vi "GXML Versioning.vi"() -> ()   [LabVIEW 2009]
doc: "This example demonstrates how to implement versioning with GXML."
uses:
  _subVIis/GXML SearchParser/gxml_SearchParser.vi
panel:
  out "Config Info v2.0":T1
  out "XML String Out":string
  in  "ConfigInfo v1.0":T2={"Enable"=TRUE, "Sample Rate"=51200.0, "Description"="Acquisition 1"}
  # "This example shows how an application can use GXML versioning to determine which type definition should be used to parse the XML string and how data from older versions can be updated to the current version.\n\nIn this example a configuration is written using an older cluster type definition (version 1.0).  The consuming\napplication however is expecting to parse its data using the current type definition (version 2.0)."
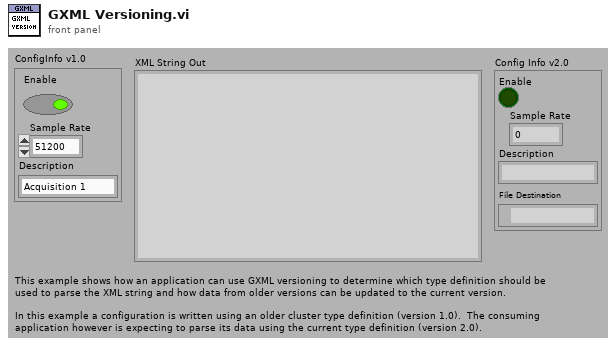
[diagram p1: front panel]
types:
  T1 = cluster{"Enable":bool, "Sample Rate":dbl, "Description":string, "File Destination":path}
  T2 = cluster{"Enable":bool, "Sample Rate":dbl, "Description":string}
  T3 = cluster{"Enable":bool, "Sample Rate":dbl, "Description":string, "Path":path}
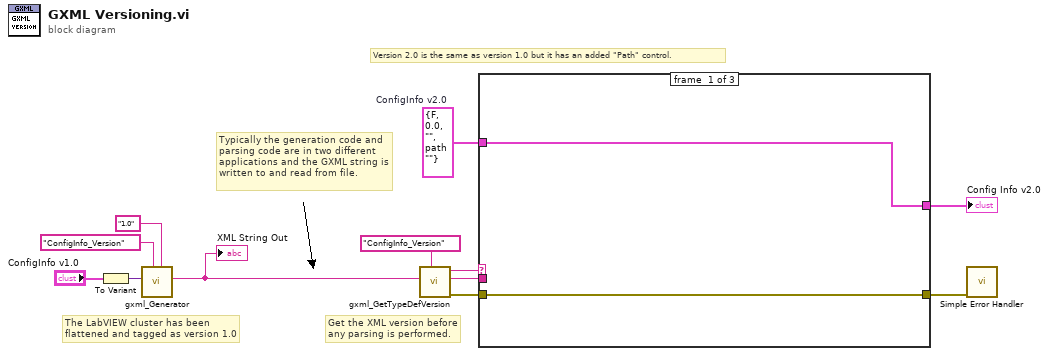
[diagram p0: block diagram]
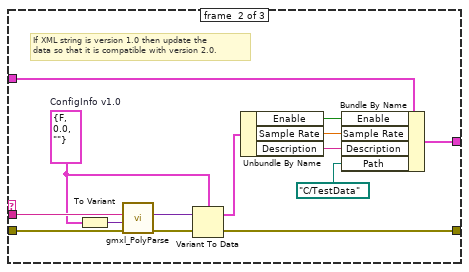
[diagram p2: hidden frame]
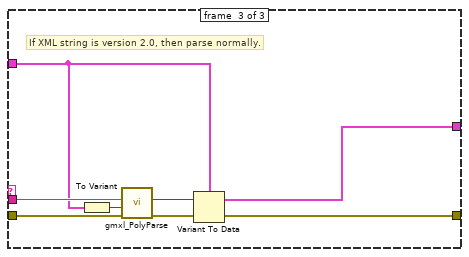
[diagram p3: hidden frame]
diagram:
  w5 = T3 {"Enable"=FALSE, "Sample Rate"=0.0, "Description"="", "Path"=path ""}  # ConfigInfo v2.0
  # "Typically the generation code and parsing code are in two different applications and the GXML string is written to and read from file."
  # "The LabVIEW cluster has been\nflattened and tagged as version 1.0"
  # "Get the XML version before\nany parsing is performed."
  # "Version 2.0 is the same as version 1.0 but it has an added \"Path\" control."
  n1 = To Variant(anything="ConfigInfo v1.0") -> (Variant=w9:variant)
  n2 = call "gxml_Generator.vi"("Version String"="1.0", "Version Tag Name"="ConfigInfo_Version", "Variant"=w9) -> ("XML String Out"=w1:string)  [unwired: 7 in, 1 out]
  "XML String Out" <- w1
  n3 = call "gxml_GetTypeDefVersion.vi"("Version Tag Name"="ConfigInfo_Version", "XML String In"=w1) -> ("error out"=w4:errorcluster, "XML String Out"=w12:string, "Version String"=w7:string)  [unwired: 7 in]
  n4 = case shown="\"1.0\"" w7 {
    tunnel: w12 -> [_ w28 w32]
    tunnel: w4 -> [w13 w27 w33]
    tunnel: [w14 w16 w31] -> w6
    tunnel: w5 -> [w14 w21 w30]
    tunnel: [w13 w15 w29] -> w3
    frame #0 {
    }
    frame #1 {
      w22 = T2 {"Enable"=FALSE, "Sample Rate"=0.0, "Description"=""}  # ConfigInfo v1.0
      # "If XML string is version 1.0 then update the\ndata so that it is compatible with version 2.0."
      n5 = To Variant(anything=w22) -> (Variant=w26:variant)
      n6 = call-poly "gmxl_PolyParse.vi"("error in"=w27, "TypeDesc"=w26, "XML String In"=w28) -> ("error out"=w25:errorcluster, "Parsed Data"=w24:variant)  [unwired: 7 in]
      n7 = Variant To Data(error in=w25, Variant=w24, type=w22) -> (error out=w15:errorcluster, data=w23:T2)
      n8 = Unbundle By Name(w23) -> ("Enable"=w20:bool, "Sample Rate"=w19:dbl, "Description"=w18:string)
      n9 = Bundle By Name(cluster=w21, "Enable"=w20, "Sample Rate"=w19, "Description"=w18, "Path"=path "C:/TestData" ("Path Destination")) -> (w16:T3)
    }
    frame #2 {
      # "If XML string is version 2.0, then parse normally."
      n10 = To Variant(anything=w30) -> (Variant=w36:variant)
      n11 = call-poly "gmxl_PolyParse.vi"("error in"=w33, "TypeDesc"=w36, "XML String In"=w32) -> ("error out"=w35:errorcluster, "Parsed Data"=w34:variant)  [unwired: 7 in]
      n12 = Variant To Data(error in=w35, Variant=w34, type=w30) -> (error out=w29:errorcluster, data=w31:T3)
    }
  }
  "Config Info v2.0" <- w6
  n13 = call <vilib>:"Simple Error Handler.vi"("error in (no error)"=w3) -> ()  [unwired: 4 in, 5 out]
